vi "experiment_finished.vi"(8 "error in (no error)":errorcluster, 11 "DL090430TriggeredExperimentController in":refnum<class "ExperimentControllerDL090803Triggered.lvclass">) -> (0 "error out":errorcluster, 3 "DL090430TriggeredExperimentController out":refnum<class "ExperimentControllerDL090803Triggered.lvclass">)   [LabVIEW 2010, in "ExperimentControllerDL090803Triggered.lvclass"]
uses:
  ExperimentControllerDL090803Triggered.lvclass
  Instrument/GenericInstrument/GenericInstrument/GenericInstrument.lvclass
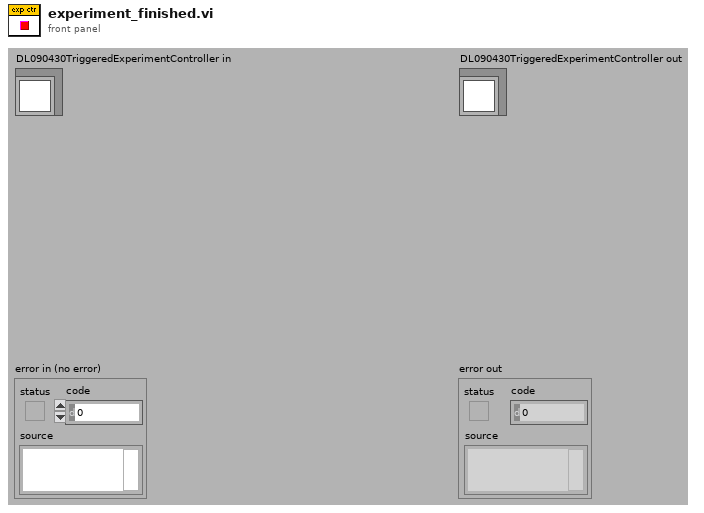
[diagram p1: front panel]
types:
  T1 = typedef "GenericToplevelComponent.lvclass/common_trigger_enum.ctl" = enum16{"NULL", "initialise", "terminate", "fetch command", "fetch data", "attach observer", "register as observer", "detach observer", "acknowledge", "start", "stop", "sweep started", "sweep finished", "experiment started", "experiment stopped"}
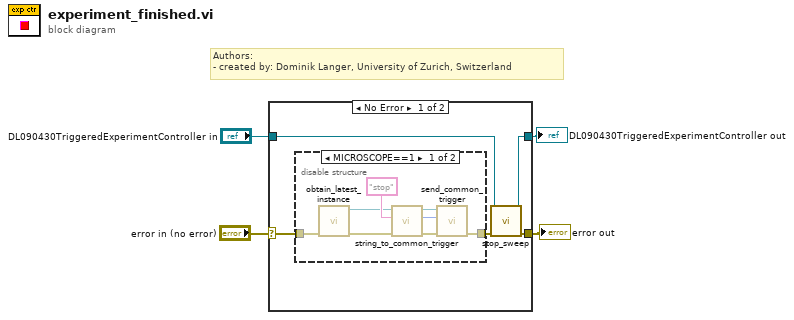
[diagram p0: block diagram]
diagram:
  # "Authors: \n- created by: Dominik Langer, University of Zurich, Switzerland"
  n1 = case shown="No Error" "error in (no error)" {
    selector: "error in (no error)" -> [w9 w20]
    tunnel: [w8 w20] -> w3
    tunnel: [w5 w19] -> w1
    tunnel: "DL090430TriggeredExperimentController in" -> [w6 w19]
    frame No Error {
      n2 = disable-structure shown="MICROSCOPE==1" {
        disable-tunnel: w9 -> [w17 w18]
        disable-tunnel: [w16 w18] -> w7
        frame condition #0 {
          n3 = call "obtain_latest_instance.vi"("error in (no error)"=w17) -> ("error out"=w14:errorcluster, "microscope"=w10:refnum<class "GenericInstrument.lvclass">)  [unwired: 9 in]
          n4 = call-dynamic "string_to_common_trigger.vi"("error in (no error)"=w14, "trigger string"="stop", "GenericToplevelComponent in"=w10) -> ("error out"=w13:errorcluster, "trigger"=w11:T1, "GenericToplevelComponent out"=w12:refnum<class "GenericInstrument.lvclass">)  [unwired: 6 in]
          n5 = call-dynamic "send_common_trigger.vi"("error in (no error)"=w13, "trigger"=w11, "GenericToplevelComponent in"=w12) -> ("error out"=w16:errorcluster)  [unwired: 6 in, 2 out]
        }
        frame condition #1 (active) {
        }
      }
      n6 = call-dynamic "stop_sweep.vi"("error in (no error)"=w7, "DL090430TriggeredExperimentController in"=w6) -> ("error out"=w8:errorcluster, "DL090430TriggeredExperimentController out"=w5:refnum<class "ExperimentControllerDL090803Triggered.lvclass">)  [unwired: 8 in]
    }
    frame Error {
    }
  }
  "error out" <- w3
  "DL090430TriggeredExperimentController out" <- w1
